vi "Script Poly VIs.vi"(8 "error in":errorcluster, 9 "Ref.Poly VIs":T1, 10 "Conpane Map":T2(c390)) -> (0 "error out":errorcluster)   [LabVIEW 2025, in "_Msg Rescript.lvlib" / "_Msg Rescript.lvclass"]
uses:
  _Msg Rescript.lvclass
  _Msg Rescript.lvclass/_Msg Rescript.ctl
  <vilib>/Utility/traverseref.llb/TRef TravTarget.ctl
  Poly VIs.ctl
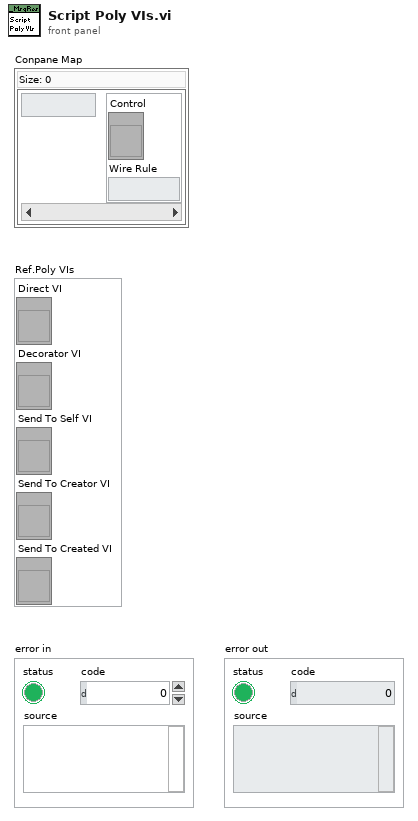
[diagram p1: front panel]
types:
  T1 = typedef "_Msg Rescript.lvlib/_Msg Rescript.lvclass/Poly VIs.ctl" = cluster{"Direct VI":refnum<vi>, "Decorator VI":refnum<vi>, "Send To Self VI":refnum<vi>, "Send To Creator VI":refnum<vi>, "Send To Created VI":refnum<vi>}
  T2 = map{i32, cluster{"Control":refnum<vi>, "Wire Rule":enum16{"Invalid Wire Rule", "Required", "Recommended", "Optional", "Dynamic Dispatch"}}}
  T3 = typedef "TRef TravTarget.ctl" = enum16{"FP", "BD", "Other"}
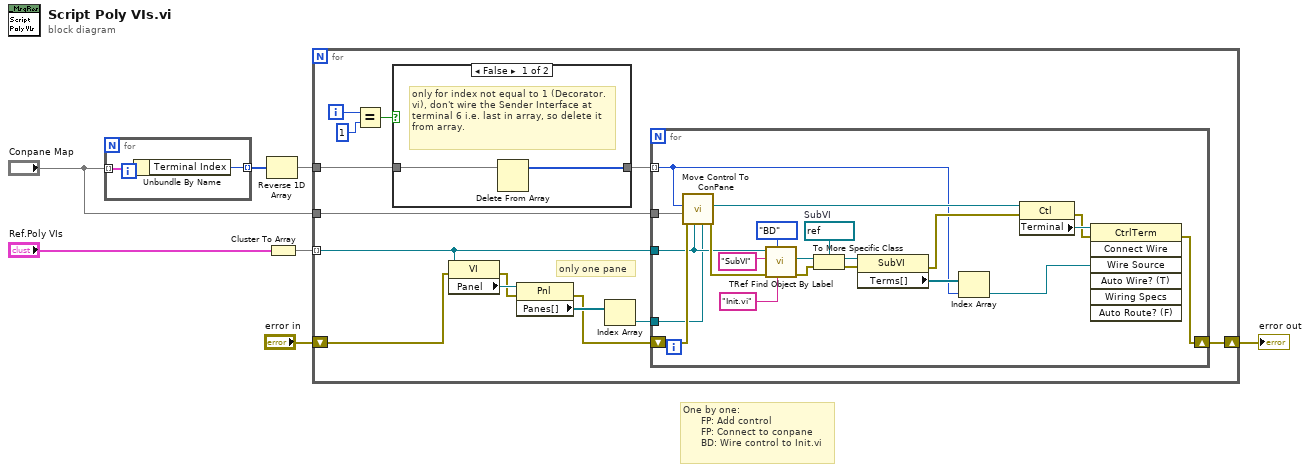
[diagram p0: block diagram]
diagram:
  # "One by one:\n      FP: Add control\n      FP: Connect to conpane\n      BD: Wire control to Init.vi"
  n1 = for {
    tunnel: "Conpane Map" -> [w9] mode=indexing
    tunnel: [w8] -> w7 mode=indexing
    n2 = Unbundle By Name(w9) -> ("Terminal Index"=w8:i32)
  }
  n3 = Reverse 1D Array(array=w7) -> (reversed array=w6:i32[])
  n4 = Cluster To Array(cluster="Ref.Poly VIs") -> (array=w1:refnum<vi>[])
  n5 = for {
    tunnel: w6 -> [w12]
    tunnel: "Conpane Map" -> [w23]
    shift-right: [w21] -> w3
    shift-left: "error in" -> [w22]
    tunnel: w1 -> [w18] mode=indexing
    i -> [w19]
    # "only one pane"
    n6 = Equal?(x=w19, y=1) -> (x = y?=w10:bool)
    n7 = case shown="False" w10 {
      tunnel: w12 -> [w25 w26]
      tunnel: [w24 w26] -> w11
      frame False {
        # "only for index not equal to 1 (Decorator.vi), don't wire the Sender Interface at terminal 6 i.e. last in array, so delete it from array."
        n8 = Delete From Array(array=w25) -> (array with subset deleted=w24:i32[])  [unwired: 2 in, 1 out]
      }
      frame True {
      }
    }
    n9 = property class="VI"(reference=w18, error in=w22) -> (error out=w15:errorcluster, "Panel"=w17:refnum<vi>)  [unwired: 1 out]
    n10 = property class="Pnl"(reference=w17, error in=w15) -> (error out=w14:errorcluster, "Panes[]"=w16:refnum<vi>[])  [unwired: 1 out]
    n11 = Index Array(array=w16) -> (element=w13:refnum<vi>)  [unwired: 1 in]
    n12 = for {
      tunnel: w11 -> [w27] mode=indexing
      tunnel: w23 -> [w28]
      tunnel: w13 -> [w29]
      tunnel: w18 -> [w30]
      shift-right: [w45] -> w21
      shift-left: w14 -> [w33]
      w43 = refnum<vi> refnum  # SubVI
      n13 = call "Move Control To ConPane.vi"("Pane"=w29, "Ref. VI"=w30, "error in"=w33, "Conpane Map"=w28, "Terminal Index"=w27) -> ("error out"=w32:errorcluster, "Control"=w31:refnum<vi>)  [unwired: 5 in]
      n14 = call <vilib>:"TRef Find Object By Label.vi"("Label"="Init.vi", "Traverse Target"=TRef_TravTarget."BD", "error in (no error)"=w32, "Class Name"="SubVI", "VI Ref"=w30) -> ("error out"=w42:errorcluster, "Found Obj Ref"=w37:refnum<vi>)  [unwired: 3 in, 2 out]
      n15 = To More Specific Class(target class=w43, reference=w37, error in=w42) -> (specific class reference=w40:refnum<vi>, error out=w39:errorcluster)
      n16 = property class="SubVI"(reference=w40, error in=w39) -> (error out=w34:errorcluster, "Terms[]"=w38:refnum<vi>[])  [unwired: 1 out]
      n17 = Index Array(array=w38, index=w27) -> (element=w35:refnum<vi>)
      n18 = property class="Ctl"(reference=w31, error in=w34) -> (error out=w46:errorcluster, "Terminal"=w47:refnum<vi>)  [unwired: 1 out]
      n19 = invoke class="CtrlTerm" method="Connect Wire"(reference=w47, error in=w46, "Wire Source"=w35) -> (error out=w45:errorcluster)  [unwired: 4 in, 6 out]
    }
  }
  "error out" <- w3
